vi "FTW-JSON-Core-EncodingFlags.vi"(0 "Indent Spaces":i32=4, 5 "Escape Unicode":bool=TRUE, 7 "Sort Keys":bool, 9 "Floating Point Significant Digits":i32=16, 11 "error in":errorcluster) -> (4 "Encoding Flags":i64 format="%016x", 15 "error out":errorcluster)   [LabVIEW 2014]
panel:
  # "Inputs"
  # "Outputs"
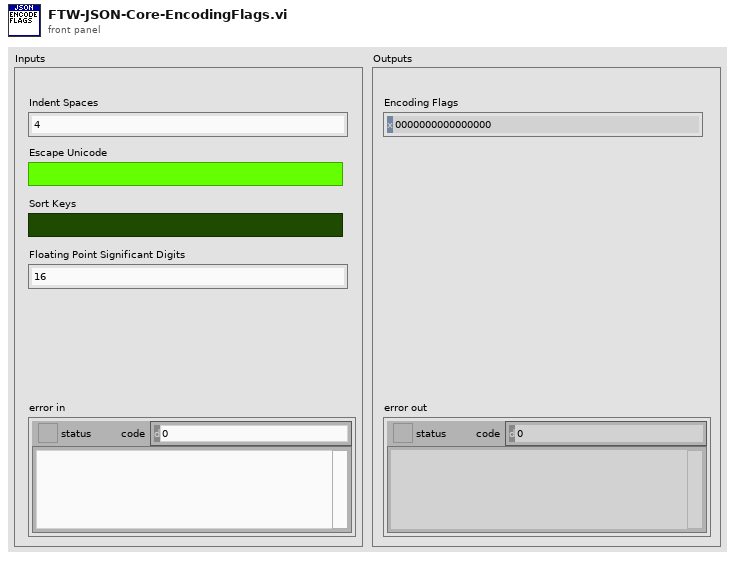
[diagram p1: front panel]
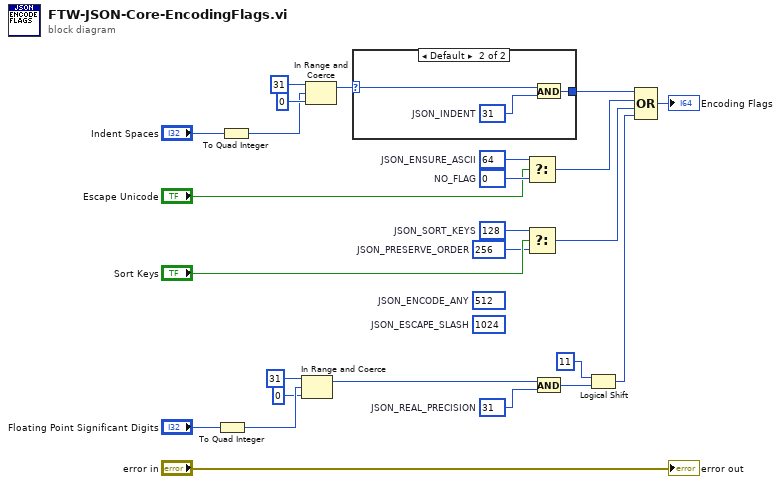
[diagram p0: block diagram]
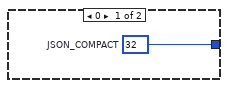
[diagram p2: hidden frame]
diagram:
  w10 = i64 31  # JSON_REAL_PRECISION
  w13 = i64 0  # NO_FLAG
  (unwired) i64 1024  # JSON_ESCAPE_SLASH
  (unwired) i64 512  # JSON_ENCODE_ANY
  w17 = i64 256  # JSON_PRESERVE_ORDER
  w18 = i64 128  # JSON_SORT_KEYS
  w14 = i64 64  # JSON_ENSURE_ASCII
  n1 = To Quad Integer(1:"Floating Point Significant Digits") -> (0:w7:i64)
  n2 = To Quad Integer(1:"Indent Spaces") -> (0:w15:i64)
  n3 = In Range and Coerce(upper limit=i64 31, x=w7, lower limit=i64 0) -> (coerced(x)=w3:i64)  [unwired: 1 out]
  n4 = In Range and Coerce(upper limit=i64 31, x=w15, lower limit=i64 0) -> (coerced(x)=w21:i64)  [unwired: 1 out]
  n5 = case shown="Default" w21 {
    selector: w21 -> [_ w27]
    tunnel: [w26 w28] -> w20
    frame 0 {
      w26 = i64 32  # JSON_COMPACT
    }
    frame Default {
      w29 = i64 31  # JSON_INDENT
      n6 = And(x=w27, y=w29) -> (x .and. y?=w28:i64)
    }
  }
  n7 = Select(t=w14, s="Escape Unicode", f=w13) -> (s? t:f=w11:i64)
  n8 = Select(t=w18, s="Sort Keys", f=w17) -> (s? t:f=w16:i64)
  n9 = And(x=w3, y=w10) -> (x .and. y?=w9:i64)
  n10 = Logical Shift(y=i16 11, x=w9) -> (x << y=w2:i64)
  n11 = Compound Arithmetic op=OR(w20, w11, w16, w2) -> (→"Encoding Flags":i64)
  "error out" <- "error in"
